vi "JTAG Init.vi"(8 "error in (no error)":errorcluster, 11 "Power Target Device":bool) -> (0 "error out":errorcluster, 3 "Device Vcc":i32)   [LabVIEW 2009]
panel:
  in  "PC start address":u16=12544 format="%04x"
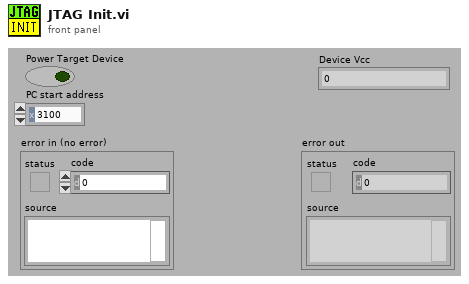
[diagram p1: front panel]
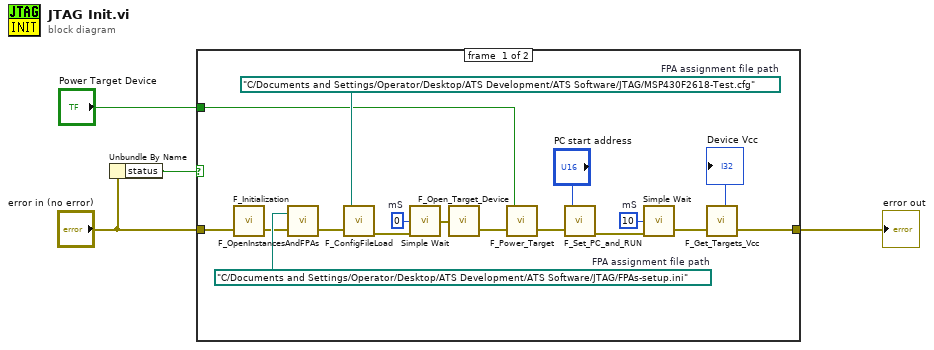
[diagram p0: block diagram]
diagram:
  n1 = Unbundle By Name("error in (no error)") -> ("status"=w4:bool)
  n2 = case shown="False" w4 {
    tunnel: [w16 w22] -> w2
    tunnel: "error in (no error)" -> [w17 w22]
    tunnel: "Power Target Device" -> [w11 _]
    frame #0 {
      w12 = u32 0  # mS
      w15 = u32 10  # mS
      w20 = path "C:/Documents and Settings/Operator/Desktop/ATS Development/ATS Software/JTAG/MSP430F2618-Test.cfg"  # FPA assignment file path
      w21 = path "C:/Documents and Settings/Operator/Desktop/ATS Development/ATS Software/JTAG/FPAs-setup.ini"  # FPA assignment file path
      n3 = call "F_Initialization.vi"("error in (no error)"=w17) -> ("error out"=w18:errorcluster)
      n4 = call "F_OpenInstancesAndFPAs.vi"("error in (no error)"=w18, "FPA assignment file path"=w21) -> ("error out"=w13:errorcluster)  [unwired: 1 out]
      n5 = call "F_ConfigFileLoad.vi"("error in (no error)"=w13, "Config file path"=w20) -> ("error out"=w9:errorcluster)  [unwired: 1 in]
      n6 = call "Simple Wait.vi"("mS"=w12, "error in"=w9) -> ("error out"=w10:errorcluster)  [unwired: 12 in, 1 out]
      n7 = call "F_Open_Target_Device.vi"("error in (no error)"=w10) -> ("error out"=w6:errorcluster)
      n8 = call "F_Power_Target.vi"("error in (no error)"=w6, "Power Target Device"=w11) -> ("error out"=w5:errorcluster)  [unwired: 1 in]
      n9 = call "F_Set_PC_and_RUN.vi"("error in (no error)"=w5, "PC start address"="PC start address") -> ("error out"=w7:errorcluster)  [unwired: 1 in]
      n10 = call "Simple Wait.vi"("mS"=w15, "error in"=w7) -> ("error out"=w14:errorcluster)  [unwired: 12 in, 1 out]
      n11 = call "F_Get_Targets_Vcc.vi"("error in (no error)"=w14) -> ("error out"=w16:errorcluster, "Device Vcc"=→"Device Vcc":i32)  [unwired: 1 in]
    }
    frame #1 {
    }
  }
  "error out" <- w2
